vi "Task3.vi"() -> ()   [LabVIEW 2017]
panel:
  out "Numeric":dbl
  out "8bit number":i16(slide) scale=0.0..255.0
  in  "8bit switches":bool[](array[boolean])
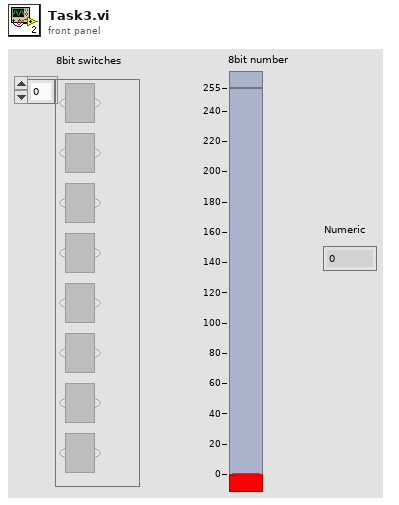
[diagram p1: front panel]
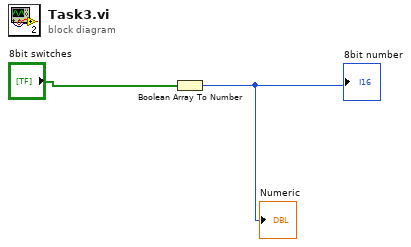
[diagram p0: block diagram]
diagram:
  n1 = Boolean Array To Number(Boolean array="8bit switches") -> (number=→"8bit number" →"Numeric":u32)
